vi "BOS_EOS.vi"() -> ()   [LabVIEW 2018, in "6509.lvlib"]
uses:
  Libraries/6509/6509.lvlib
panel:
  out "appended array":bool[](array[boolean])
  out "edge_type":T1(ring)
  in  "edge_curr":cluster{"itrp":bool[], "time":dbl}
  in  "edge_prev":cluster{"itrp":bool[], "time":dbl}
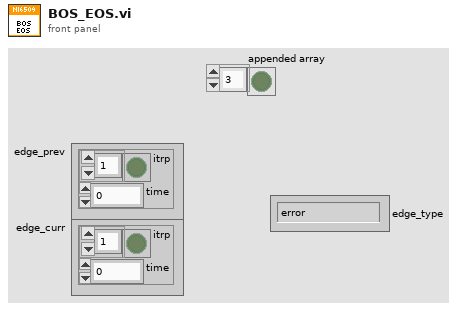
[diagram p1: front panel]
types:
  T1 = enum16{"error", "bos_rise", "bos_fall", "eos_rise", "eos_fall"}
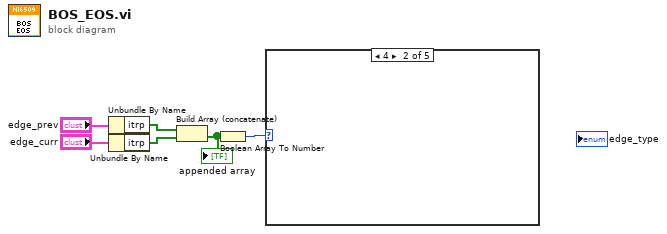
[diagram p0: block diagram]
diagram:
  n1 = Unbundle By Name("edge_prev") -> ("itrp"=w3:bool[])
  n2 = Unbundle By Name("edge_curr") -> ("itrp"=w2:bool[])
  n3 = Build Array (concatenate)(w3, w2) -> (w1:bool[])
  "appended array" <- w1
  n4 = Boolean Array To Number(Boolean array=w1) -> (number=w6:u32)
  n5 = case shown="4" w6 {
    frame Default {
    }
    frame 4 {
    }
    frame 1 {
    }
    frame 8 {
    }
    frame 2 {
    }
  }
